vi "generate_DAC_voltages_rearranged2.vi"(7 "focus mode?":bool, 8 "derived values":T1, 9 "scan specification":T4={"x amplitude"=0, "x resolution (pixels)"=0, "x offset fly-forward (iterations)"=0, "x offset fly-back (iterations)"=0, "y resolution (nr. of lines)"=0, "y step size"=0, "iterations per pixel"=0, "number of frames"=0, "y offset (pixels)"=0, "number of y-brake lines  (before y-fly-back)"=0, "number y-brake lines (after y-fly-back)"=0, "number of y-fly-back steps"=8, "lines per z step"=0, "number of z/intensity tuples"=0, "number of repetitions (volumes or planes)"=0, "z step size derived"=0, "choose the beginning of z scan"=FALSE, "number of frames (settings)"=0, "FPGA trajectory?"=FALSE}, 10 "counter cluster in":T2, 11 "resonant trigger":bool) -> (0 "acquire?":bool, 1 "fly-back acquisition phase?":bool, 2 "counter cluster out":T2, 3 "DAC voltages":T3 {"ch6" max=4095 step=1; "ch5" max=4095 step=1; "ch4" max=4095 step=1; "ch3" max=4095 step=1; "ch2" max=4095 step=1; "ch1" max=4095 step=1; "ch0" max=4095 step=1})   [LabVIEW 2010]
uses:
  scan_specification_cluster.ctl
  common_typedefs/DAC_voltage_cluster.ctl
  counter_cluster.ctl
  derived_values_cluster.ctl
panel:
  out "co":u16
  out "integer":u16
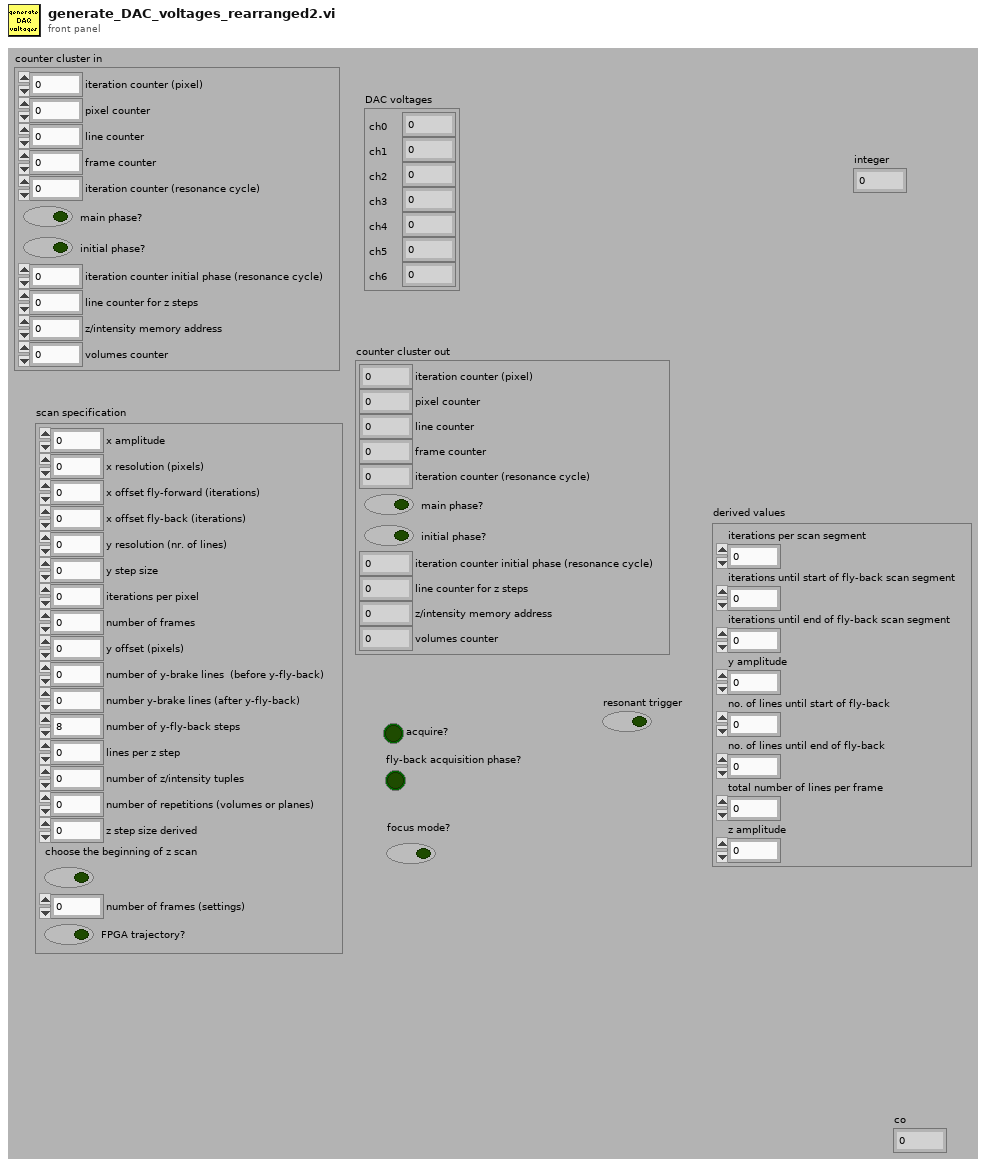
[diagram p1: front panel]
types:
  T1 = typedef "derived_values_cluster.ctl" = cluster{"iterations per scan segment":u16, "iterations until start of fly-back scan segment":u16, "iterations until end of fly-back scan segment":u16, "y amplitude":u16, "no. of lines until start of fly-back":u16, "no. of lines until end of fly-back":u16, "total number of lines per frame ":u16, "z amplitude":u16}
  T2 = typedef "counter_cluster.ctl" = cluster{"iteration counter (pixel)":u16, "pixel counter":u16, "line counter":u16, "frame counter":u16, "iteration counter (resonance cycle)":u16, "main phase?":bool, "initial phase?":bool, "iteration counter initial phase (resonance cycle)":u16, "line counter for z steps":u16, "z/intensity memory address":u32, "volumes counter":u16}
  T3 = typedef "DAC_voltage_cluster.ctl" = cluster{"ch0":u16, "ch1":i16, "ch2":i16, "ch3":u16, "ch4":u16, "ch5":u16, "ch6":u16}
  T4 = typedef "scan_specification_cluster.ctl" = cluster{"x amplitude":u16, "x resolution (pixels)":u16, "x offset fly-forward (iterations)":u16, "x offset fly-back (iterations)":u16, "y resolution (nr. of lines)":u16, "y step size":u16, "iterations per pixel":u16, "number of frames":i32, "y offset (pixels)":u16, "number of y-brake lines  (before y-fly-back)":u16, "number y-brake lines (after y-fly-back)":u16, "number of y-fly-back steps":u16, "lines per z step":u16, "number of z/intensity tuples":u16, "number of repetitions (volumes or planes)":i32, "z step size derived":u16, "choose the beginning of z scan":bool, "number of frames (settings)":i32, "FPGA trajectory?":bool}
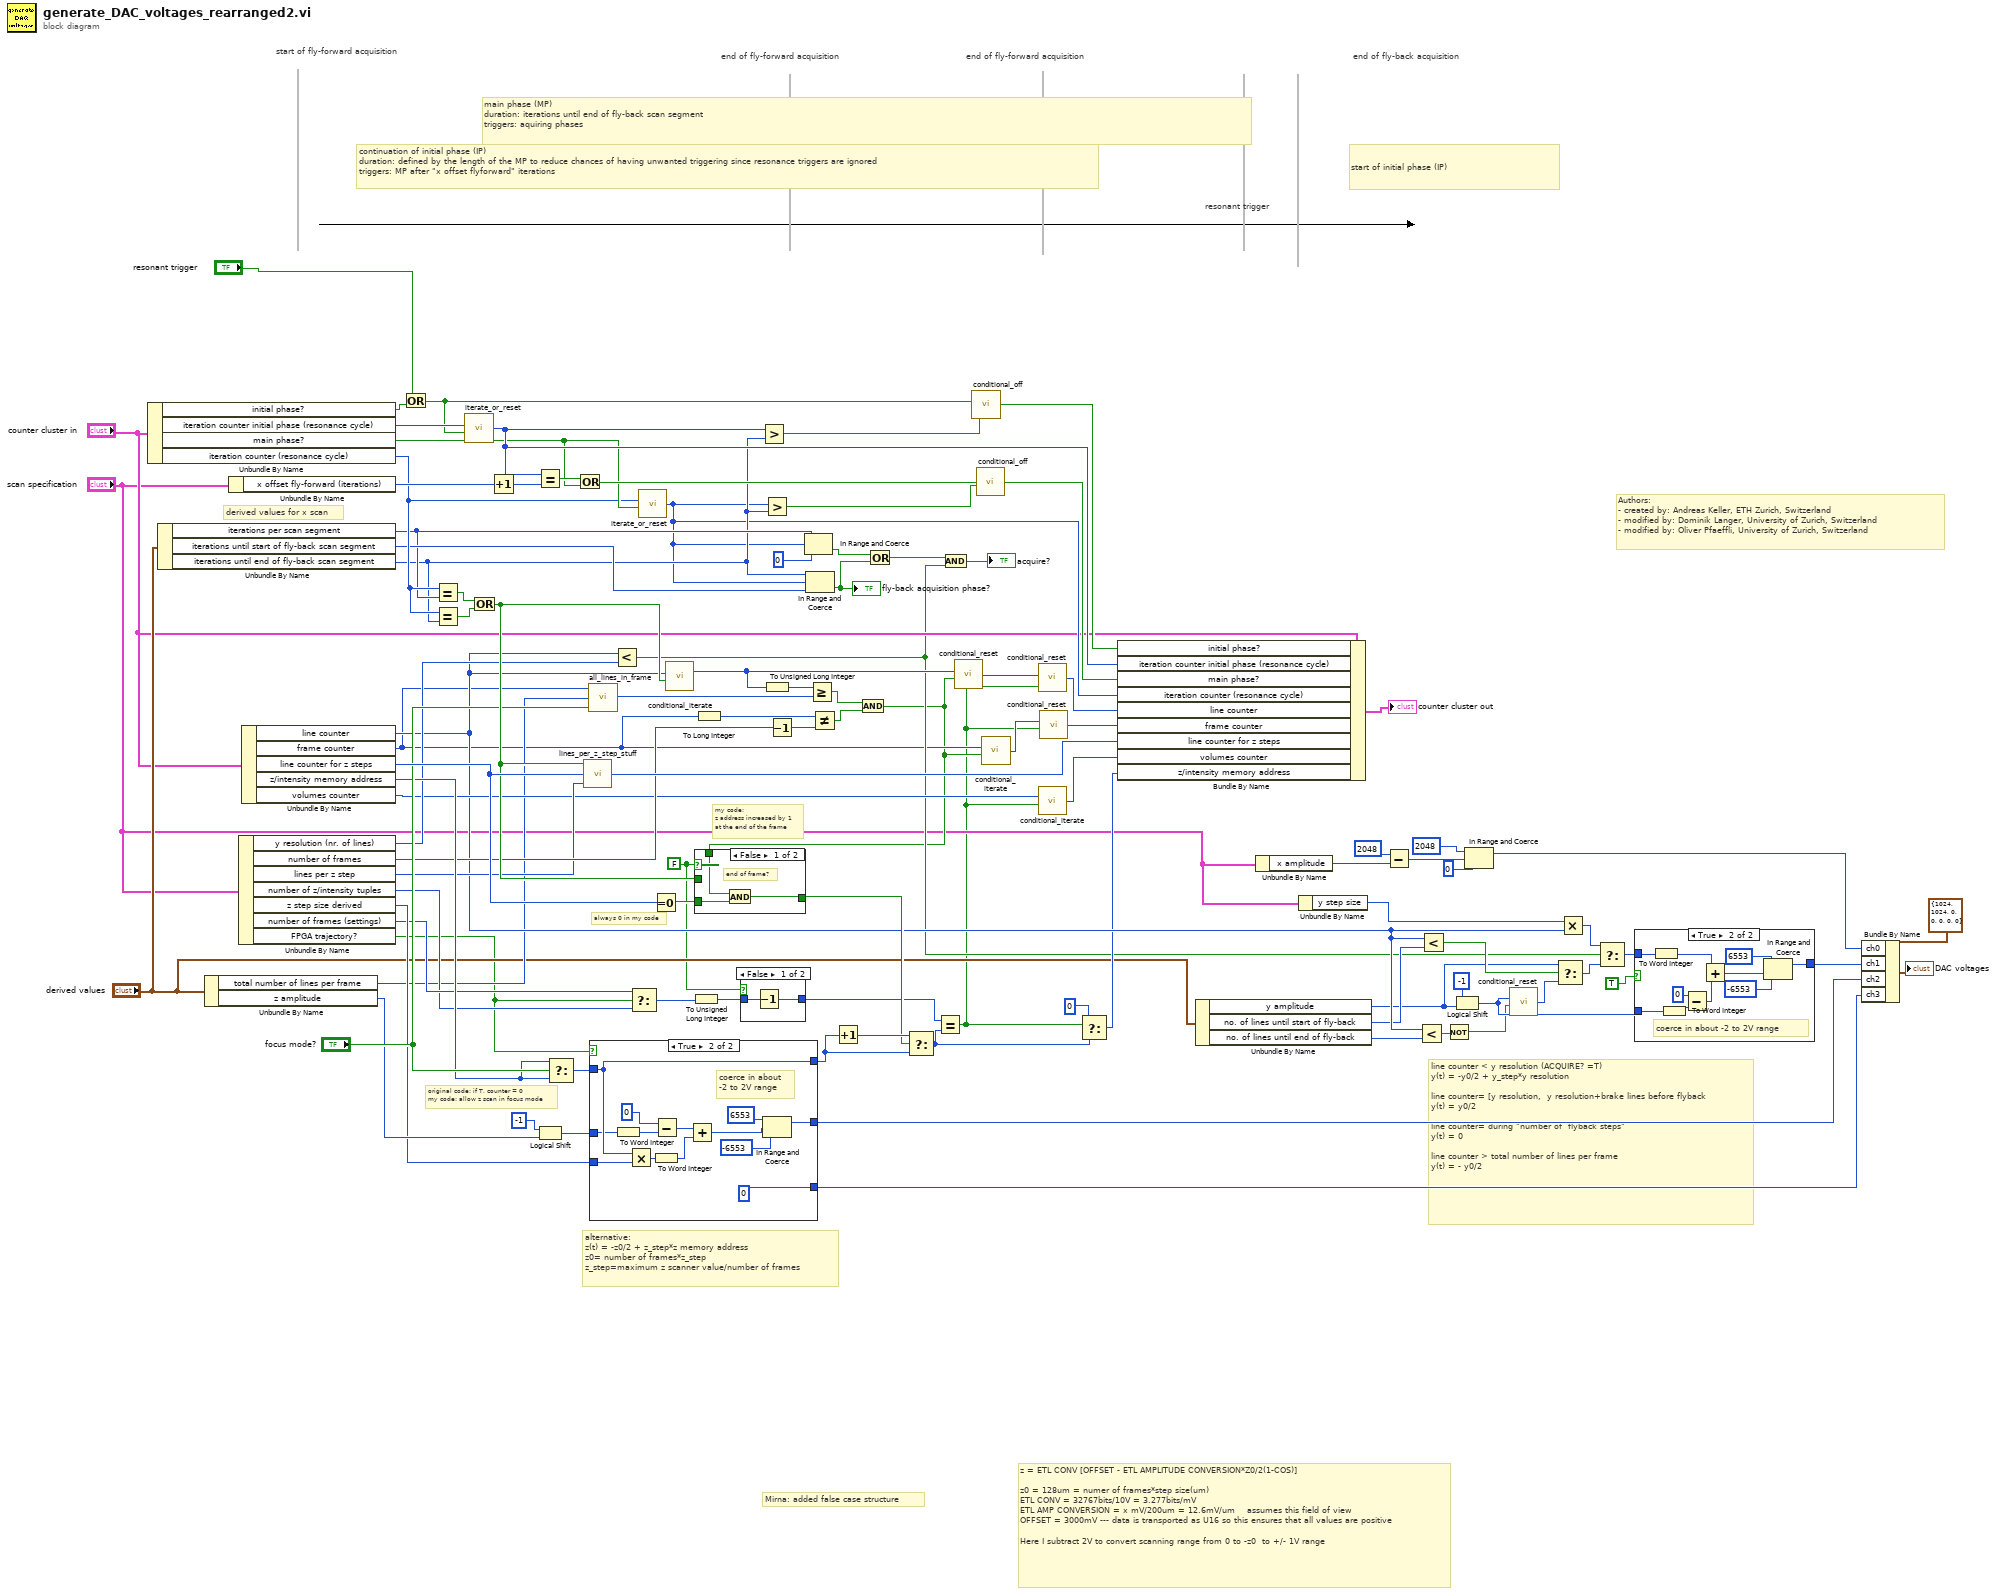
[diagram p0: block diagram]
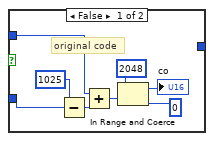
[diagram p3: hidden frame]
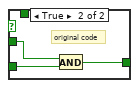
[diagram p4: hidden frame]
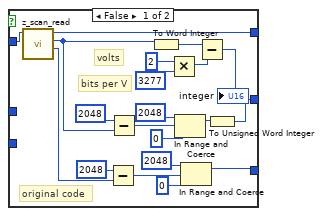
[diagram p5: hidden frame]
diagram:
  w3 = FALSE
  # "always 0 in my code"
  # "line counter < y resolution (ACQUIRE? =T)\ny(t) = -y0/2 + y_step*y resolution\n\nline counter= [y resolution,  y resolution+brake lines before flyback\ny(t) = y0/2\n\nline counter= during \"number of  flyback steps\"\ny(t) = 0\n\nline counter > total number of lines per frame\ny(t) = - y0/2"
  # "derived values for x scan"
  # "z = ETL CONV [OFFSET - ETL AMPLITUDE CONVERSION*Z0/2(1-COS)]\n\nz0 = 128um = numer of frames*step size(um)\nETL CONV = 32767bits/10V = 3.277bits/mV\nETL AMP CONVERSION = x mV/200um = 12.6mV/um    assumes this field of view\nOFFSET = 3000mV --- data is transported as U16 so this ensures that all values are positive\n\nHere I subtract 2V to convert scanning range from 0 to -z0  to +/- 1V range"
  # "my code:\nz address increased by 1\nat the end of the frame"
  # "alternative:\nz(t) = -z0/2 + z_step*z memory address\nz0= number of frames*z_step\nz_step=maximum z scanner value/number of frames"
  # "original code: if T, counter = 0\nmy code: allow z scan in focus mode"
  # "Mirna: added false case structure"
  # "start of initial phase (IP)"
  # "continuation of initial phase (IP)\nduration: defined by the length of the MP to reduce chances of having unwanted triggering since resonance triggers are ignored\ntriggers: MP after \"x offset flyforward\" iterations"
  # "end of fly-back acquisition"
  # "end of fly-forward acquisition"
  # "end of fly-forward acquisition"
  # "start of fly-forward acquisition"
  # "main phase (MP)\nduration: iterations until end of fly-back scan segment\ntriggers: aquiring phases"
  # "resonant trigger"
  # "Authors: \n- created by: Andreas Keller, ETH Zurich, Switzerland\n- modified by: Dominik Langer, University of Zurich, Switzerland\n- modified by: Oliver Pfaeffli, University of Zurich, Switzerland"
  n1 = Unbundle By Name("counter cluster in") -> ("initial phase?"=w37:bool, "iteration counter initial phase (resonance cycle)"=w36:u16, "main phase?"=w35:bool, "iteration counter (resonance cycle)"=w34:u16)
  n2 = Unbundle By Name("derived values") -> ("iterations per scan segment"=w30:u16, "iterations until start of fly-back scan segment"=w31:u16, "iterations until end of fly-back scan segment"=w29:u16)
  n3 = Unbundle By Name("derived values") -> ("total number of lines per frame"=w18:u16, "z amplitude"=w52:u16)
  n4 = Unbundle By Name("scan specification") -> ("x offset fly-forward (iterations)"=w38:u16)
  n5 = Unbundle By Name("scan specification") -> ("y resolution (nr. of lines)"=w26:u16, "number of frames"=w27:i32, "lines per z step"=w24:u16, "number of z/intensity tuples"=w41:u16, "z step size derived"=w51:u16, "number of frames (settings)"=w42:i32, "FPGA trajectory?"=w12:bool)
  n6 = Unbundle By Name("counter cluster in") -> ("line counter"=w22:u16, "frame counter"=w8:u16, "line counter for z steps"=w77:u16, "z/intensity memory address"=w56:u32, "volumes counter"=w23:u16)
  n7 = Or(x="resonant trigger", y=w37) -> (x .or. y?=w33:bool)
  n8 = Equal?(x=w34, y=w30) -> (x = y?=w79:bool)
  n9 = Equal?(x=w34, y=w29) -> (x = y?=w80:bool)
  n10 = call "iterate_or_reset.vi"("iterate?"=w33, "number in"=w36) -> ("number out"=w49:u16)  [unwired: 4 in]
  n11 = Or(x=w79, y=w80) -> (x .or. y?=w72:bool)
  n12 = Increment(x=w38) -> (x+1=w32:u16)
  n13 = Equal?(x=w49, y=w32) -> (x = y?=w86:bool)
  n14 = Logical Shift(y=i16 -1 ("n"), x=w52) -> (x << y=w62:u16)
  n15 = Select(t=w56, s="focus mode?", f=w56) -> (s? t:f=w57:u32)
  n16 = Or(x=w86, y=w35) -> (x .or. y?=w61:bool)
  n17 = call "lines_per_z_step_stuff.vi"("lines per z step"=w24, "line counter for z steps"=w77, ">end of line?>"=w72) -> ("number out"=w78:u16)
  n18 = call "all_lines_in_frame.vi"("focus mode?"="focus mode?", "total number of lines per frame"=w18, "frame counter"=w8) -> ("Numeric"=w25:u32)
  n19 = case shown="True" w12 {
    tunnel: [w114 u16 0 ("intensity")] -> w59
    tunnel: [w121 w131] -> w71
    tunnel: [w106 w122] -> w58
    tunnel: w57 -> [w120 w131]
    tunnel: w62 -> [_ w123]
    tunnel: w51 -> [_ w132]
    frame False {
      # "bits per V"
      # "volts"
      # "original code"
      n20 = call "z_scan_read.vi"("address in"=w120) -> ("intensity"=w117:u16, "z-value"=w102:i16, "address out"=w121:u32)  [unwired: 8 in]
      n21 = Subtract(x=i16 2048, y=w117) -> (x-y=w113:u16)
      n22 = Subtract(x=i16 2048, y=w102) -> (x-y=w109:i16)
      n23 = To Word Integer(number=w102) -> (16bit integer=w107:i16)
      n24 = Multiply(x=i16 2 ("y"), y=i16 3277) -> (x*y=w104:i16)
      n25 = In Range and Coerce(upper limit=i16 2048, x=w109, lower limit=i16 0) -> (coerced(x)=w110:i16)  [unwired: 1 out]
      n26 = In Range and Coerce(upper limit=u16 2048, x=w113, lower limit=u16 0) -> (coerced(x)=w114:u16)  [unwired: 1 out]
      n27 = Subtract(x=w107, y=w104) -> (x-y=w106:i16)
      n28 = To Unsigned Word Integer(number=w110) -> (unsigned 16bit integer=→"integer":u16)
    }
    frame True {
      # "coerce in about\n-2 to 2V range"
      n29 = To Word Integer(number=w123) -> (16bit integer=w128:i16)
      n30 = Multiply(x=w131, y=w132) -> (x*y=w129:u32)
      n31 = To Word Integer(number=w129) -> (16bit integer=w127:i16)
      n32 = Subtract(x=i16 0, y=w128) -> (x-y=w130:i16)
      n33 = Add(x=w130, y=w127) -> (x+y=w124:i16)
      n34 = In Range and Coerce(upper limit=i16 6553, x=w124, lower limit=i16 -6553) -> (coerced(x)=w122:i16)  [unwired: 1 out]
    }
  }
  n35 = Less?(x=w22, y=w26) -> (x < y?=w9:bool)
  n36 = Select(t=w42, s=w12, f=w41) -> (s? t:f=w55:i32)
  n37 = call "iterate_or_reset.vi"("iterate?"=w35, "number in"=w34) -> ("number out"=w28:u16)  [unwired: 4 in]
  n38 = Equal To 0?(x=w77) -> (x = 0?=w73:bool)
  n39 = call "conditional_iterate.vi"("iterate?"=w72, "number in"=w22) -> ("number out"=w19:u16)  [unwired: 4 in]
  n40 = To Unsigned Long Integer(number=w55) -> (unsigned 32bit integer=w2:u32)
  n41 = To Long Integer(number=w8) -> (32bit integer=w65:i32)
  n42 = case shown="False" w3 {
    tunnel: w2 -> [w136 w137]
    tunnel: [w135 w137] -> w1
    frame False {
      n43 = Decrement(x=w136) -> (x-1=w135:u32)
    }
    frame True {
    }
  }
  n44 = Greater?(x=w49, y=w29) -> (0:w81:bool)
  n45 = Greater?(x=w28, y=w29) -> (0:w84:bool)
  n46 = To Unsigned Long Integer(number=w19) -> (unsigned 32bit integer=w40:u32)
  n47 = Decrement(x=w27) -> (x-1=w66:i32)
  n48 = In Range and Coerce(upper limit=w30, x=w28, lower limit=u16 0) -> (In Range?=w96:bool)  [unwired: 1 out]
  n49 = In Range and Coerce(upper limit=w29, x=w28, lower limit=w31) -> (In Range?=w43:bool)  [unwired: 1 out]
  "fly-back acquisition phase?" <- w43
  n50 = Greater Or Equal?(x=w40, y=w25) -> (x >= y?=w67:bool)
  n51 = Not Equal?(x=w65, y=w66) -> (x != y?=w39:bool)
  n52 = Increment(x=w71) -> (x+1=w76:u32)
  n53 = And(x=w67, y=w39) -> (x .and. y?=w7:bool)
  n54 = case shown="False" w3 {
    tunnel: w73 -> [w140 w143]
    tunnel: w72 -> [_ w142]
    tunnel: [w139 w141] -> w50
    tunnel: w7 -> [w138 _]
    frame False {
      # "end of frame?"
      n55 = And(x=w138, y=w140) -> (x .and. y?=w139:bool)
    }
    frame True {
      # "original code"
      n56 = And(x=w142, y=w143) -> (x .and. y?=w141:bool)
    }
  }
  n57 = Or(x=w96, y=w43) -> (x .or. y?=w90:bool)
  n58 = Select(t=w76, s=w50, f=w71) -> (s? t:f=w75:u32)
  n59 = Equal?(x=w1, y=w75) -> (x = y?=w4:bool)
  n60 = And(x=w90, y=w9) -> (x .and. y?=→"acquire?":bool)
  n61 = call "conditional_reset.vi"("reset?"=w7, "number in"=w19) -> ("number out"=w69:u16)  [unwired: 4 in]
  n62 = call "conditional_off.vi"("switch off?"=w81, "boolean in"=w33) -> ("boolean out"=w85:bool)  [unwired: 4 in]
  n63 = call "conditional_off.vi"("switch off?"=w84, "boolean in"=w61) -> ("boolean out"=w83:bool)  [unwired: 4 in]
  n64 = call "conditional_iterate.vi"("iterate?"=w7, "number in"=w8) -> ("number out"=w53:u16)  [unwired: 4 in]
  n65 = call "conditional_reset.vi"("reset?"=w4, "number in"=w69) -> ("number out"=w68:u16)  [unwired: 4 in]
  n66 = call "conditional_iterate.vi"("iterate?"=w4, "number in"=w23) -> ("number out"=w70:u16)  [unwired: 4 in]
  n67 = call "conditional_reset.vi"("reset?"=w4, "number in"=w53) -> ("number out"=w54:u16)  [unwired: 4 in]
  n68 = Select(t=u32 0, s=w4, f=w75) -> (s? t:f=w21:u32)
  n69 = Bundle By Name(cluster="counter cluster in", "initial phase?"=w85, "iteration counter initial phase (resonance cycle)"=w49, "main phase?"=w83, "iteration counter (resonance cycle)"=w28, "line counter"=w68, "frame counter"=w54, "line counter for z steps"=w78, "volumes counter"=w70, "z/intensity memory address"=w21) -> (→"counter cluster out":T2)
  n70 = Unbundle By Name("derived values") -> ("y amplitude"=w13:u16, "no. of lines until start of fly-back"=w15:u16, "no. of lines until end of fly-back"=w16:u16)
  n71 = Unbundle By Name("scan specification") -> ("x amplitude"=w20:u16)
  n72 = Unbundle By Name("scan specification") -> ("y step size"=w5:u16)
  n73 = Subtract(x=u16 2048, y=w20) -> (x-y=w94:u16)
  n74 = Less?(x=w22, y=w16) -> (x < y?=w89:bool)
  n75 = Less?(x=w22, y=w15) -> (x < y?=w101:bool)
  n76 = Not(x=w89) -> (.not. x?=w44:bool)
  n77 = Logical Shift(y=i16 -1 ("n"), x=w13) -> (x << y=w45:u16)
  n78 = In Range and Coerce(upper limit=u16 2048, x=w94, lower limit=u16 0) -> (coerced(x)=w93:u16)  [unwired: 1 out]
  n79 = call "conditional_reset.vi"("reset?"=w44, "number in"=w45) -> ("number out"=w82:u16)  [unwired: 4 in]
  n80 = Select(t=w13, s=w101, f=w82) -> (s? t:f=w46:u16)
  n81 = Multiply(x=w5, y=w22) -> (x*y=w14:u16)
  n82 = Select(t=w14, s=w9, f=w46) -> (s? t:f=w48:u16)
  n83 = case shown="True" TRUE {
    tunnel: [_ w154] -> w60
    tunnel: w45 -> [w144 w153]
    tunnel: w48 -> [w145 w152]
    frame False {
      # "original code"
      n84 = Subtract(x=u16 1025, y=w144) -> (x-y=w147:u16)
      n85 = Add(x=w145, y=w147) -> (x+y=w146:u16)
      n86 = In Range and Coerce(upper limit=u16 2048, x=w146, lower limit=u16 0) -> (coerced(x)=→"co":u16)  [unwired: 1 out]
    }
    frame True {
      # "coerce in about -2 to 2V range"
      n87 = To Word Integer(number=w152) -> (16bit integer=w158:i16)
      n88 = To Word Integer(number=w153) -> (16bit integer=w159:i16)
      n89 = Subtract(x=i16 0, y=w159) -> (x-y=w160:i16)
      n90 = Add(x=w158, y=w160) -> (x+y=w155:i16)
      n91 = In Range and Coerce(upper limit=i16 6553, x=w155, lower limit=i16 -6553) -> (coerced(x)=w154:i16)  [unwired: 1 out]
    }
  }
  n92 = Bundle By Name(cluster=T3 {"ch0"=1024, "ch1"=1024, "ch2"=0, "ch3"=0, "ch4"=0, "ch5"=0, "ch6"=0} ("DAC voltage"), "ch0"=w93, "ch1"=w60, "ch2"=w58, "ch3"=w59) -> (→"DAC voltages":T3)
